vi "lanelog2.vi"(6 "xsensor":T1={"idx"=1, "x"=-35.60561147, "y"=-90.69379038, "h"=0.8330275943157105, "x_path"=0.0}, 7 "thresh":dbl=0.02, 8 "lane_log":dbl[][](array[numeric])=array7715x4[30860 elements], 9 "sensor":dbl[][](array[numeric])=[[-3.0874260564438702, 8.254219212686142, 0.33125647926136603, -1.2, 268.0], [-3.251465137645852, 8.1435734553204, 0.33125647926136603, -1.2, 284.0], [-3.2918636404136175, 8.115022616326533, 0.33125647926136603, -1.2, 272.0], [-3.2146540135510326, 8.265920567763587, 0.3295810856706975, -1.2, 268.0], [-3.0941669932632254, 8.356869302518275, 0.3293716614718639, -1.2, 216.0], [-3.0675596258112376, 8.409121589077968, 0.32874338887536325, -1.2, 248.0], [-3.1950142718158414, 8.327140005961258, 0.32874338887536325, -1.2, 236.0], [-3.278772864980552, 8.270644121512921, 0.32874338887536325, -1.2, 248.0], [-2.9865656875850273, 8.47047999653983, 0.3285339646765297, -1.2, 232.0], [-3.035050878170219, 8.452752896063785, 0.3283245404776961, -1.2, 204.0], [-2.9543519196681682, 8.617087628303914, 0.32623029848936036, -1.2, 224.0], [-2.998893873836392, 8.591111528384989, 0.32623029848936036, -1.2, 196.0], [-2.9033727279755284, 8.737823052620522, 0.3245549048986918, -1.2, 216.0], [-2.968662847780547, 8.747093819694697, 0.3237172081033576, -1.2, 192.0], [-2.9052595387814195, 8.85082243489861, 0.32246066291035613, -1.2, 188.0], [-2.734592721427704, 8.98474447764757, 0.32162296611502184, -1.2, 204.0], [-2.791429232542248, 8.978488337161597, 0.3212041177173547, -1.2, 224.0], [-2.839131166422159, 8.953920226823765, 0.3212041177173547, -1.2, 196.0], [-2.886616889471603, 8.928936779344951, 0.3212041177173547, -1.2, 216.0], [-2.6987125748878515, 9.157968574659893, 0.3186910273313519, -1.2, 196.0], [-2.765515279987869, 9.17014660250537, 0.3178533305360176, -1.2, 220.0], [-2.6830373985326297, 9.253792269139186, 0.3170156337406833, -1.2, 220.0], [-4.28548337639476, 9.508026110543323, 0.39847829900104376, -0.3999999999999999, 204.0], [6.270261138102536, 8.950654849997015, 0.2759684907693037, -1.2, 308.0], [6.263336924153402, 9.139533897307718, 0.27345540038330085, -1.2, 304.0], [6.193207282056716, 9.275259222095512, 0.27261770358796655, -1.2, 312.0], [6.091471855365504, 9.38246599277969, 0.27261770358796655, -1.2, 324.0], [6.4696355580106255, 9.02559077208453, 0.2717800067926323, -1.2, 240.0], [6.372215345218233, 9.137659907105647, 0.2717800067926323, -1.2, 256.0], [6.331823345079176, 9.30204711946733, 0.2701046132019638, -1.2, 264.0], [6.072715111455862, 9.572715111455864, 0.2701046132019638, -1.2, 332.0], [6.258607904594664, 9.439197138421996, 0.2692669164066295, -1.2, 276.0], [6.182525166787418, 9.57555056054587, 0.2684292196112952, -1.2, 276.0], [6.049147437675454, 9.764075544301484, 0.2675915228159609, -1.2, 328.0], [6.0207247852542345, 9.956436871376717, 0.2650784324299581, -1.2, 324.0], [6.215701669208983, 9.825143971096239, 0.2642407356346238, -1.2, 276.0], [6.104366004380429, 9.932659572856856, 0.2642407356346238, -1.2, 280.0], [6.045206253694134, 10.097184975373532, 0.2625653420439552, -1.2, 284.0], [5.987405501886605, 10.149687481752428, 0.2625653420439552, -1.2, 332.0], [6.008645752931635, 10.291538564175015, 0.2600522516579524, -1.2, 288.0], [5.949150359744033, 10.34371462365704, 0.2600522516579524, -1.2, 332.0], [5.967118589360381, 10.48659821129467, 0.2575391612719496, -1.2, 292.0], [5.905922582465032, 10.538404455235977, 0.2575391612719496, -1.2, 332.0], [5.845104223695827, 10.718102585492996, 0.25544491928361385, -1.2, 344.0], [5.742861784006737, 10.85052788528084, 0.2546072224882796, -1.2, 352.0], [5.946027011549364, 10.713107553966188, 0.25418837409061246, -1.2, 296.0], [5.685904682379038, 11.045450364978343, 0.2520941321022767, -1.2, 352.0], [5.893920691194497, 10.90967382499498, 0.2516752837046096, -1.2, 296.0], [5.812396612769266, 11.074862742777189, 0.24999989011394105, -1.2, 300.0], [5.635624312811938, 11.256771414722133, 0.24916219331860678, -1.2, 340.0], [5.750674853192741, 11.271591029935388, 0.24748679972793824, -1.2, 300.0], [5.545267703886312, 11.419463018156659, 0.24748679972793824, -1.2, 340.0], [5.462116471720623, 11.597920686443521, 0.24539255773960256, -1.2, 344.0], [5.683835103994589, 11.468442930129942, 0.24497370934193538, -1.2, 284.0], [5.566552204276135, 11.599383715798275, 0.2441360125466011, -1.2, 284.0], [5.51264120473925, 11.828692341891706, 0.240785225365264, -1.2, 288.0], [5.439750670877296, 11.876481469970823, 0.240785225365264, -1.2, 336.0], [5.303328472257424, 11.987099673000078, 0.24036637696759688, -1.2, 344.0], [-1.928655864366284, 13.422074272450256, 0.2382721349792612, -1.2, 324.0], [5.216191450902815, 12.181200407749735, 0.23785328658159402, -1.2, 348.0], [5.473882232873657, 12.092273991781463, 0.23659674138859263, -1.2, 284.0], [5.323092676171175, 12.186497764352836, 0.23659674138859263, -1.2, 296.0], [5.153869423312828, 12.426763696753529, 0.23408365100258977, -1.2, 340.0], [5.2721670641556875, 12.450363583742815, 0.2324082574119212, -1.2, 288.0], [-1.900299672338241, 13.75309951845401, 0.23157056061658696, -1.2, 296.0], [-1.8211698834585328, 13.82836765049368, 0.2303140154235855, -1.2, 372.0], [5.174236572168083, 12.645432179932216, 0.2298951670259184, -1.2, 288.0], [5.103925680397715, 12.70772566679367, 0.22947631862825127, -1.2, 344.0], [5.017550333081534, 12.936639702633745, 0.22612553144691414, -1.2, 344.0], [5.147413862635719, 12.980356990567492, 0.22403128945857842, -1.2, 288.0], [8.180852483152144, 10.611506567635107, 0.3743231383700968, -0.3999999999999999, 264.0], [4.942872250794322, 13.200933006778827, 0.22193704747024273, -1.2, 348.0], [5.055038418263844, 13.210638452637436, 0.2206805022772413, -1.2, 288.0], [-1.8068749197163638, 14.297458756228902, 0.2206805022772413, -1.2, 308.0], [8.174393871184286, 10.860257301297807, 0.373206136722423, -0.3999999999999999, 256.0], [8.132454974984348, 11.083636951508186, 0.37236838548666756, -0.3999999999999999, 264.0], [4.974014493298352, 13.47632967793971, 0.21649201830056994, -1.2, 288.0], [4.886766302989657, 13.51935572391995, 0.21649201830056994, -1.2, 308.0], [8.02763653917211, 11.252198494109617, 0.3720891350747491, -0.3999999999999999, 284.0], [8.41805715455429, 10.9476678431101, 0.37153063425091215, -0.3999999999999999, 212.0], [-1.762629762368157, 14.628806331963263, 0.2139789279145671, -1.2, 312.0], [8.004253700261659, 11.50425370026166, 0.37097213342707525, -0.3999999999999999, 304.0], [8.353148660757368, 11.154250519053866, 0.37090232082409563, -0.3999999999999999, 220.0], [8.218291344725634, 11.298867285084208, 0.37090232082409563, -0.3999999999999999, 236.0], [8.622793513388025, 10.864561394524376, 0.370832508221116, -0.3999999999999999, 176.0], [7.974483755589461, 11.757819665743355, 0.36985513177940144, -0.3999999999999999, 320.0], [8.202180279054376, 11.560260111808223, 0.3697155065734422, -0.3999999999999999, 248.0], [4.954095970806885, 13.886478196863694, 0.20895274714256143, -1.2, 248.0], [4.880170386307381, 13.965559166701984, 0.20811505034722713, -1.2, 260.0], [7.945087273837262, 12.020062990878387, 0.36866831752874796, -0.3999999999999999, 368.0], [8.263518845062517, 11.909017868700095, 0.3676909410870333, -0.3999999999999999, 256.0], [8.115502673534229, 12.051955424034883, 0.3676909410870333, -0.3999999999999999, 296.0], [-1.7422907602406512, 15.157939689347018, 0.20308886957522146, -1.2, 264.0], [7.929004456398092, 12.306051579412163, 0.36727206546915564, -0.3999999999999999, 392.0], [7.774110039342803, 12.443090583519641, 0.36727206546915564, -0.3999999999999999, 412.0], [4.917183201802519, 14.28977377780451, 0.20162290018338652, -1.2, 224.0], [8.052839027989592, 12.288131688987452, 0.36678337724829835, -0.3999999999999999, 348.0], [4.891968691273311, 14.487541577387939, 0.19806268880321581, -1.2, 260.0], [7.771112819957454, 12.761251621639218, 0.36559656299764487, -0.3999999999999999, 416.0], [8.030759275666764, 12.57712212750872, 0.365387125188706, -0.3999999999999999, 360.0], [-1.6961480258098567, 15.568720307529205, 0.19471190162187874, -1.2, 296.0], [7.949050394089805, 12.807142204926757, 0.3645493739529506, -0.3999999999999999, 372.0], [7.7089869232088795, 13.01980603123654, 0.364479561349971, -0.3999999999999999, 424.0], [7.566295141983507, 13.184416153684932, 0.36420031093805255, -0.3999999999999999, 448.0], [4.907524501146654, 14.786533649341463, 0.19219881123587584, -1.2, 304.0], [7.938062739362771, 13.129640127422718, 0.36287387148143985, -0.3999999999999999, 380.0], [7.76879334061014, 13.266711783841115, 0.36287387148143985, -0.3999999999999999, 396.0], [7.516486463232196, 13.474714437812196, 0.36280405887846023, -0.3999999999999999, 456.0], [4.902600205433592, 15.049802292658747, 0.18717263046387017, -1.2, 300.0], [7.411791406878046, 13.701455690730548, 0.3619663076427049, -0.3999999999999999, 468.0], [7.6945569471755055, 13.527741846330688, 0.361756869833766, -0.3999999999999999, 424.0], [7.278507600876223, 13.894786122248709, 0.3614078068188679, -0.3999999999999999, 480.0], [7.5659614658398775, 13.724810089569369, 0.3611983690099291, -0.3999999999999999, 432.0], [7.163086529840346, 14.119712503220669, 0.36057005558311256, -0.3999999999999999, 492.0], [-1.6742837675349664, 16.217447813122682, 0.18130875289653026, -1.2, 288.0], [7.456044248361615, 13.952988517530661, 0.3603606177741737, -0.3999999999999999, 440.0], [4.939359591017299, 15.424668914071585, 0.17963335930586166, -1.2, 276.0], [7.340445944696752, 14.180415124015806, 0.3595228665384183, -0.3999999999999999, 456.0], [4.910015355954023, 15.652714457593937, 0.1754448753291903, -1.2, 272.0], [-2.0742704566937493, 16.596428237795855, 0.35742848844902986, -0.3999999999999999, 244.0], [7.351621486160834, 14.60708847142727, 0.3570096128311522, -0.3999999999999999, 460.0], [-1.6314726207982264, 16.787278211536382, 0.16958099776185032, -1.2, 292.0], [6.947694316000941, 15.062905099763684, 0.3558227985804987, -0.3999999999999999, 576.0], [4.950345642278116, 16.06718454758031, 0.16706790737584754, -1.2, 240.0], [7.3285880609769, 15.003578979950875, 0.35477560953580445, -0.3999999999999999, 476.0], [4.940810185204615, 16.371250584204297, 0.16120402980850757, -1.2, 248.0], [7.377499944938261, 15.538985731940056, 0.3514246045927829, -0.3999999999999999, 480.0], [4.971854164908072, 16.797828014132726, 0.15261763765633118, -1.2, 220.0], [4.975301680149189, 17.169529021184545, 0.14528779069715625, -1.2, 228.0], [-1.5383215259591212, 18.136151645750907, 0.1417275793169856, -1.2, 172.0], [1.6829626062501868, 18.271173220882176, 0.13858621633448204, -1.2, 76.0], [4.982643392608833, 17.570550880741774, 0.13732967114148065, -1.2, 208.0], [-1.1993764728960121, 18.73952302036782, 0.12979039998347214, -1.2, 436.0], [4.9833552728263575, 17.972714590665475, 0.129371551585805, -1.2, 192.0], [1.621925956717769, 18.9315946699765, 0.12497364341030004, -1.2, 236.0], [-1.4948658186201547, 19.024775107896094, 0.1232982498196315, -1.2, 172.0], [4.9710734881443015, 18.356972582706735, 0.12183228042779648, -1.2, 184.0], [10.1762046864033, 15.52061845794352, 0.5599548496928946, 0.40000000000000013, 412.0], [4.4892978065922735, 18.655615402218494, 0.1189003416441265, -1.2, 392.0], [10.116711660579657, 15.882236625148431, 0.5616303521644053, 0.40000000000000013, 432.0], [4.423009309038194, 18.924866549582596, 0.11387416087212082, -1.2, 424.0], [4.9679034872117604, 18.789634776867167, 0.1132458882756201, -1.2, 180.0], [10.208563049778917, 16.21960594386651, 0.563864355459753, 0.40000000000000013, 388.0], [-1.4211984035446172, 19.7443720851159, 0.10842913170244806, -1.2, 224.0], [4.9154615434653435, 19.08985228247094, 0.1075914349071137, -1.2, 216.0], [4.802613585016308, 19.208641220118103, 0.10591604131644522, -1.2, 268.0], [-1.86214748615549, 19.843858727865292, 0.3351582680985325, -0.3999999999999999, 500.0], [4.41648153671134, 19.425317939974306, 0.10382179932810948, -1.2, 440.0], [10.245755173166765, 16.496678478471168, 0.5655398579312637, 0.40000000000000013, 396.0], [10.13194907010119, 16.585593551005047, 0.5655398579312637, 0.40000000000000013, 424.0], [8.89513720681148, 17.59793922259855, 0.5663776091670192, 0.40000000000000013, 364.0], [-1.803072050702221, 20.655084627603436, 0.3295732598601633, -0.3999999999999999, 420.0], [-1.4600881893088467, 22.052179466228814, 0.32007874585493556, -0.3999999999999999, 508.0], [-1.6254149910617555, 22.078578361528226, 0.3197994954430171, -0.3999999999999999, 368.0], [-0.876993498557809, 23.58645347846649, 0.02884793614569159, -1.2, 264.0], [-1.7323054850638269, 24.34764225753624, 0.5960479654333557, 0.40000000000000013, 184.0], [4.576693870008543, 24.144131958105543, 0.0070678194670003025, -1.2, 164.0], [-1.7766743936812326, 24.881605315546707, 0.8994243306968406, 1.2000000000000006, 212.0], [-15.383269013420207, 18.88326901342021, -0.005707056661847398, -1.2, 172.0], [-15.516925908799797, 18.748440622546504, -0.005707056661847398, -1.2, 176.0], [-15.663784770939868, 18.62634112429063, -0.006125905059514547, -1.2, 156.0], [-15.867710423236526, 18.557894946543833, -0.00822014704785018, -1.2, 132.0], [1.9091635206414816, 25.321838895456125, -0.008848419644350902, -1.2, 340.0], [-15.161125487767853, 19.4764927159004, -0.011361510030353794, -1.2, 164.0], [-1.6392398550297682, 25.55863652788837, 0.6044254777909096, 0.40000000000000013, 188.0], [4.639571181211605, 25.327466274196635, -0.017434811796527283, -1.2, 172.0], [-0.7857642968418002, 26.001345425033872, -0.02162329577319866, -1.2, 236.0], [0.19726369493970786, 26.104180522661046, -0.023508113562700772, -1.2, 208.0], [3.9287964216078732, 25.781311718843845, -0.02392696196036792, -1.2, 224.0], [-1.6774482452010537, 26.072792518250637, 0.9241363861592018, 1.2000000000000006, 220.0], [1.1851494290302318, 26.1139982507089, -0.024345810358035125, -1.2, 212.0], [2.989699229479819, 26.209020218132554, -0.02979083952770789, -1.2, 252.0], [2.7914143198272865, 26.23424524468249, -0.02979083952770789, -1.2, 116.0], [-0.0, 26.424971072078208, -0.03020968792537504, -1.2, 84.0], [5.3831189045097885, 25.922303935324, 0.2890121375290067, -0.3999999999999999, 244.0], [-1.5343200205313599, 26.909199859587602, 0.6137803665901781, 0.40000000000000013, 200.0], [4.702058107639062, 26.6113539682675, -0.04403168504839061, -1.2, 160.0], [-1.5981019113415127, 27.882323464453414, 0.9618327419492443, 1.2000000000000006, 180.0], [16.87235585354733, 21.43584249865242, 0.965811801727082, 1.2000000000000006, 236.0], [-0.6472139558002346, 28.216103807544194, -0.06790604371541759, -1.2, 80.0], [16.912004682939006, 21.79530359253437, 0.9718851034932556, 1.2000000000000006, 276.0], [4.761548009355336, 27.996040933764434, -0.07272280028858963, -1.2, 136.0], [16.966816300178685, 22.179008023982007, 0.97858667785593, 1.2000000000000006, 252.0], [17.14934975532431, 22.71422306055236, 0.9894767361952754, 1.2000000000000006, 192.0], [17.0667193182793, 22.960863590383795, 0.9921992507801118, 1.2000000000000006, 72.0], [5.438837287934404, 29.087717665370338, 0.26737023060532583, -0.3999999999999999, 140.0], [5.5183699426079125, 30.623654823461283, 0.2567587149524243, -0.3999999999999999, 136.0], [5.594383409940466, 32.280607638486906, 0.24530944806376734, -0.3999999999999999, 136.0], [2.3560692275628514, 33.43669797801458, 0.24035275325221464, -0.3999999999999999, 200.0], [5.663742107532391, 34.05881781210548, 0.23302242993935499, -0.3999999999999999, 128.0], [15.696846843198209, 30.963785907053047, 1.1126181651094145, 1.2000000000000006, 216.0], [15.945986127827634, 30.8430340000858, 1.1130370135070815, 1.2000000000000006, 212.0], [15.47612601588197, 31.13461144760037, 1.1134558619047488, 1.2000000000000006, 220.0], [-1.573164496371527, 36.25144044389028, 0.6789155251701594, 0.40000000000000013, 176.0], [-1.2951497592364731, 36.463762582363366, 0.6803117772297517, 0.40000000000000013, 180.0], [5.758033248807259, 36.15542928071491, 0.21850140851959496, -0.3999999999999999, 128.0], [10.0910638783173, 35.998536724162264, 0.6875722879396318, 0.40000000000000013, 264.0], [-0.8195652580345191, 41.06014402087102, 0.7122859493944156, 0.40000000000000013, 236.0], [6.04917334542589, 41.692977372214614, 0.18003466427782683, -0.3999999999999999, 120.0], [6.247751551440067, 45.30468176887548, 0.15490212720516522, -0.3999999999999999, 84.0], [10.576764453944458, 46.723668750702885, 0.7606660832592892, 0.40000000000000013, 160.0], [18.29351193435394, 44.11009062363429, 1.382984805803553, 1.2000000000000006, 164.0], [10.286262869518918, 47.1841965407068, 0.7633189621725146, 0.40000000000000013, 148.0], [6.550718221917733, 50.11078209610396, 0.12139207777494981, -0.3999999999999999, 40.0], [10.924256810644076, 51.77826832915608, 0.795572384749097, 0.40000000000000013, 160.0], [-1.7372882317377514, 18.747983116378037, 0.12853385479047075, -1.2, 120.0], [11.262063566611518, 15.06083163069632, 0.5626775412090995, 0.40000000000000013, 100.0], [8.976613577038671, 17.86558466119368, 0.33173745055253134, -0.3999999999999999, 160.0], [8.96290906479165, 18.71600016117027, 0.32671094313799903, -0.3999999999999999, 164.0], [-2.155816147837948, 21.05771354301394, 0.3265015053290602, -0.3999999999999999, 380.0], [9.024780067116186, 19.131377603380102, 0.323988251621794, -0.3999999999999999, 156.0], [9.045600358828692, 19.48804450755426, 0.3217542483264463, -0.3999999999999999, 148.0], [9.041479077757348, 19.811260034561684, 0.3197994954430171, -0.3999999999999999, 156.0], [-1.3236875014373035, 22.42961318623577, 0.05251287061388493, -1.2, 156.0], [9.07056698382929, 20.205906190633105, 0.31728624173575093, -0.3999999999999999, 156.0], [9.093442564981476, 20.602278093067493, 0.31477298802848475, -0.3999999999999999, 152.0], [5.027751135547025, 22.263822685673617, 0.04308878166637431, -1.2, 220.0], [13.677266938894665, 19.945126022164064, 0.5993291577733977, 0.40000000000000013, 108.0], [6.320922215936061, 24.174804981229045, 0.2990651523580713, -0.3999999999999999, 168.0], [-1.5122834965924712, 25.12666157030228, 0.2986462767401936, -0.3999999999999999, 292.0], [-15.18884666612654, 19.228511154290864, -0.00801072284901666, -1.2, 164.0], [-15.991197551190128, 18.41203296189243, -0.00801072284901666, -1.2, 124.0], [4.974826021189758, 25.048338889544475, -0.013246327819855908, -1.2, 136.0], [-15.18477247651323, 19.783674872656796, -0.01638769080235941, -1.2, 164.0], [-15.143410526013682, 20.02613264222062, -0.019529053784863026, -1.2, 152.0], [6.004699976609632, 25.15224862071348, 0.29313108110480396, -0.3999999999999999, 64.0], [-15.132414799181563, 20.306249255557532, -0.023717537761534402, -1.2, 152.0], [5.8672847673986706, 25.397004854406784, 0.29173482904521164, -0.3999999999999999, 120.0], [-14.882714626526145, 20.620604720041705, -0.025183507153369367, -1.2, 212.0], [-15.03791801192453, 21.107139779497775, -0.03502644449854714, -1.2, 176.0], [0.41091403159128786, 27.04124910340555, -0.04319398825305637, -1.2, 120.0], [3.8942692333612956, 26.7712353102285, -0.044241109247224186, -1.2, 92.0], [1.0339888538441397, 27.182238288137274, -0.04654477543439345, -1.2, 116.0], [3.756731756174191, 27.219070815772636, -0.053036925598234086, -1.2, 96.0], [16.668723246512226, 20.91237546586442, 0.9549217433877364, 1.2000000000000006, 160.0], [-15.042878891887115, 22.411490638873143, -0.056178288580737645, -1.2, 148.0], [0.6330815038741477, 27.676407242397655, -0.056597136978404794, -1.2, 112.0], [3.3978617547396803, 27.677042650522004, -0.06141389355157695, -1.2, 152.0], [-15.049621716930838, 22.76263738425686, -0.062042166148077615, -1.2, 148.0], [0.8538033900408014, 27.949730131020374, -0.062461014545744764, -1.2, 116.0], [3.6294029746828156, 27.784902355416687, -0.06434583233524688, -1.2, 88.0], [-15.051368401443346, 23.115325196741345, -0.06790604371541759, -1.2, 144.0], [16.331597840810588, 22.122618200125487, 0.6229258175805077, 0.40000000000000013, 156.0], [5.625888766858202, 27.868401465052543, 0.2753986799479816, -0.3999999999999999, 100.0], [-15.066143200716514, 23.4934473163024, -0.07439819387925822, -1.2, 132.0], [-15.224123706487509, 24.074222375009924, -0.08612594901393816, -1.2, 132.0], [15.388533709826934, 24.10774585394575, 0.6295580148635712, 0.40000000000000013, 60.0], [-15.18503985850474, 24.40041432288007, -0.09115212978594373, -1.2, 92.0], [15.450544583691912, 24.57188399004637, 0.6324203315857354, 0.40000000000000013, 88.0], [9.403345837579257, 27.9965534130117, 0.2668117297814889, -0.3999999999999999, 128.0], [5.703044844702137, 29.224772877763986, 0.2660437911487131, -0.3999999999999999, 64.0], [9.466886860277452, 29.510057881143965, 0.2567587149524243, -0.3999999999999999, 128.0], [15.599171906131094, 29.719850640073204, 0.6629982516908071, 0.40000000000000013, 176.0], [15.848136819476986, 29.6169211826018, 0.6632775021027255, 0.40000000000000013, 176.0], [16.228041929851543, 29.72422353746002, 0.6653020675891343, 0.40000000000000013, 148.0], [-1.0867438434896055, 34.62027195581754, 0.2326035543214773, -0.3999999999999999, 208.0], [11.202409620014603, 33.06825475520069, 0.6707474506215444, 0.40000000000000013, 132.0], [10.995870935203495, 33.30561238280741, 0.6717946396662386, 0.40000000000000013, 88.0], [10.418705939012487, 35.09571994456489, 0.682266530113181, 0.40000000000000013, 104.0], [5.888755068804653, 38.68981269103743, 0.20090863256873187, -0.3999999999999999, 128.0], [21.264902026527764, 37.86369875407095, 1.2964926116852886, 1.2000000000000006, 108.0], [21.17311499265992, 39.08880663879596, 1.3174350315686456, 1.2000000000000006, 84.0], [21.513995338753997, 38.95396704895709, 1.3186915767616472, 1.2000000000000006, 124.0], [17.080070877486495, 42.31741385340898, 0.7460752492365496, 0.40000000000000013, 156.0], [8.278950878194507, 19.403716667083884, 0.32482600285754937, -0.3999999999999999, 48.0], [-2.667894854589383, 21.35130129946067, 0.323988251621794, -0.3999999999999999, 340.0], [8.149121025638326, 20.208174144360875, 0.3202183710608948, -0.3999999999999999, 124.0], [9.120446875494231, 21.399884852746606, 0.3097464806139525, -0.3999999999999999, 152.0], [6.279426242486466, 24.69898772096905, 0.2956443348120701, -0.3999999999999999, 84.0], [9.243287120931221, 23.78254244454064, 0.29438770795843705, -0.3999999999999999, 148.0], [6.229252435277006, 25.223984917116187, 0.292223517266069, -0.3999999999999999, 60.0], [9.244898599965028, 24.264382226537055, 0.29131595342733396, -0.3999999999999999, 144.0], [-15.084549481174566, 20.549981599367705, -0.026858900744037906, -1.2, 148.0], [9.334488223102976, 24.967853172167995, 0.2865686964247201, -0.3999999999999999, 152.0], [16.333140340768534, 20.56182098917662, 0.6148973682378519, 0.40000000000000013, 100.0], [16.27269945637997, 20.798388974896767, 0.6158049320765869, 0.40000000000000013, 108.0], [11.633788245920316, 24.27362367751091, 0.6162238076944646, 0.40000000000000013, 120.0], [9.318710318537917, 25.453505750353774, 0.283496941893617, -0.3999999999999999, 144.0], [16.270457361193163, 21.101281609903406, 0.6173408093421384, 0.40000000000000013, 120.0], [16.223815690819396, 21.36102814499319, 0.6184578109898123, 0.40000000000000013, 124.0], [9.306634273479593, 25.968202683080712, 0.2802157495535751, -0.3999999999999999, 136.0], [16.213823438051257, 21.66605437803303, 0.6199936882553638, 0.40000000000000013, 136.0], [7.840406989925826, 26.93250647257559, 0.2774930580373701, -0.3999999999999999, 84.0], [8.09993828830126, 27.023928885387402, 0.27630624378671664, -0.3999999999999999, 92.0], [16.377343075265326, 22.506842263569443, 0.6251598208758554, 0.40000000000000013, 112.0], [7.736971672108107, 28.038539141289487, 0.2703721725334493, -0.3999999999999999, 76.0], [16.245694733302315, 24.864173105513157, 0.6373770263972881, 0.40000000000000013, 84.0], [9.529953587218, 30.411758734122486, 0.25068501849319774, -0.3999999999999999, 120.0], [14.563985000188746, 30.04663922418586, 0.6613925618222759, 0.40000000000000013, 188.0], [15.284129991017839, 29.70813053868281, 0.6618114374401536, 0.40000000000000013, 204.0], [15.084614101362881, 29.892600775732266, 0.6622303130580313, 0.40000000000000013, 188.0], [-1.3574022550676748, 34.58962300498183, 0.23274317952743653, -0.3999999999999999, 92.0], [9.62873489352778, 33.13419886563537, 0.23246392911551808, -0.3999999999999999, 88.0], [15.941280736440438, 32.55711784764017, 1.1442412191332834, 1.2000000000000006, 112.0], [-0.9436559897075923, 39.536768353342815, 0.19832556625848607, -0.3999999999999999, 76.0], [-0.6715522340536157, 41.97320172198243, 0.18136110373443953, -0.3999999999999999, 132.0], [-0.3541141808009181, 44.077465969623496, 0.16670045710872028, -0.3999999999999999, 104.0], [17.438697502854822, 42.21247295163448, 0.7464243122514476, 0.40000000000000013, 164.0], [17.80935122293895, 42.131469169923385, 0.7469828130752845, 0.40000000000000013, 160.0]], 11 "Lane_M":dbl[](array[numeric])=[0.8601491478953653, 0.8717844136967624, 0.882947592858927, 0.8936326403234123, 0.9038337699485205, 0.9135454576426009, 0.9227624443554423, 0.9314797389261423, 0.9396926207859084, 0.9473966425143293, 0.9545876322477319, 0.9612616959383189, 0.9674152194628639, 0.9730448705798238, 0.9781476007338057, 0.9827206467064133, 0.9867615321125792, 0.9902680687415704, 0.993238357741943, 0.9956707906498045, 0.9975640502598242, 0.9989171113385246, 0.9997292411794617, 1.0, 0.9997292411794617, 0.9989171113385246, 0.9975640502598242, 0.9956707906498045, 0.993238357741943, 0.9902680687415704, 0.9867615321125792, 0.9827206467064133]) -> (0 "lane_log_out":dbl[][](array[numeric]), 1 "sensor_out":dbl[][](array[numeric]), 2 "lane_I_out":dbl[](array[numeric]), 3 "lane_M_out":dbl[](array[numeric]), 4 "size":i32)   [LabVIEW 2012]
uses:
  G_NAV.vi
  G_SEN.vi
  <vilib>/Analysis/Matrix/Numeric/Conversions/Array To Matrix - RA2.vi
  <vilib>/Analysis/baseanly.llb/Real Inverse Matrix.vi
  <vilib>/Analysis/baseanly.llb/A x Vector.vi
  <vilib>/Analysis/NI_AALBase.lvlib
  <vilib>/Analysis/Matrix/NI_Matrix.lvlib
panel:
  out "Y":dbl[](array[numeric])
  out "X":dbl[](array[numeric])
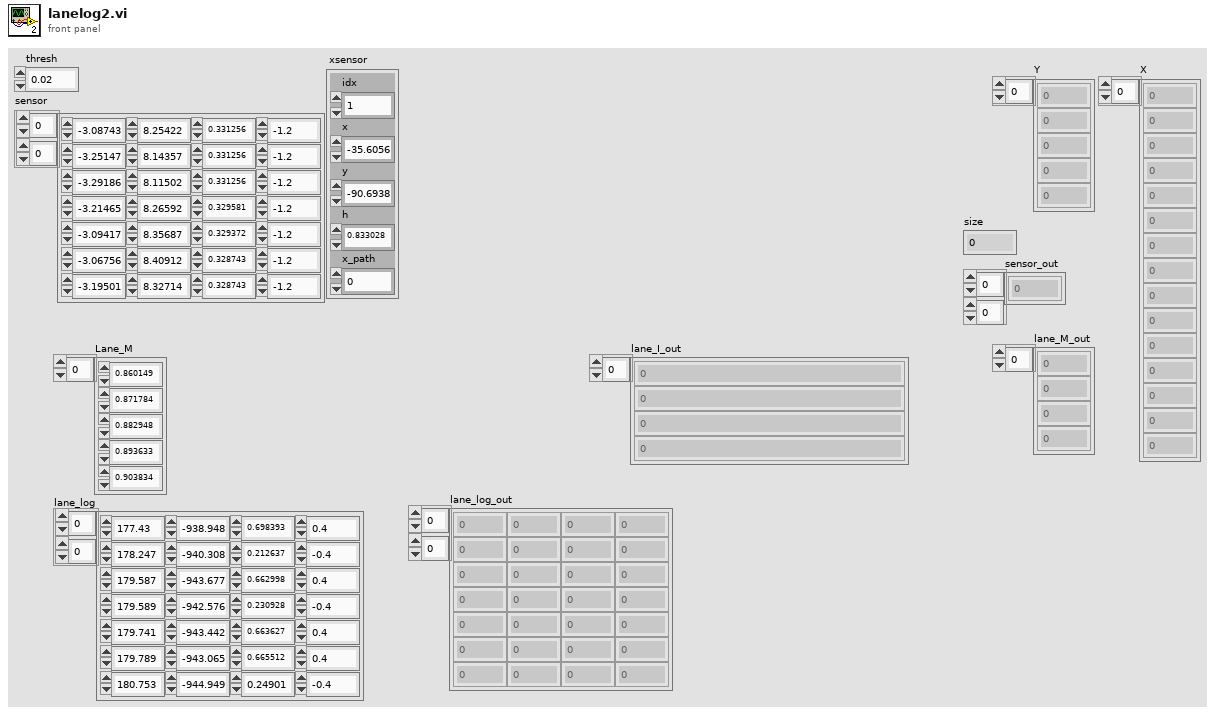
[diagram p1: front panel]
types:
  T1 = cluster{"idx":i32, "x":dbl, "y":dbl, "h":dbl, "x_path":dbl}
  T2 = cluster{"GPSTime":dbl, "attitude[2]":dbl, "lcc[0]":dbl, "lcc[1]":dbl, "heading_GPS":dbl}
  T3 = cluster{i16, "element":dbl, "element":dbl, "element":dbl, "element":dbl}[]
  T4 = cluster{i16, "Real Matrix Element":dbl, "Real Matrix Element":dbl}[]
  T5 = typedef "NI_Matrix.lvlib/RealMatrix.ctl" = dbl[][]
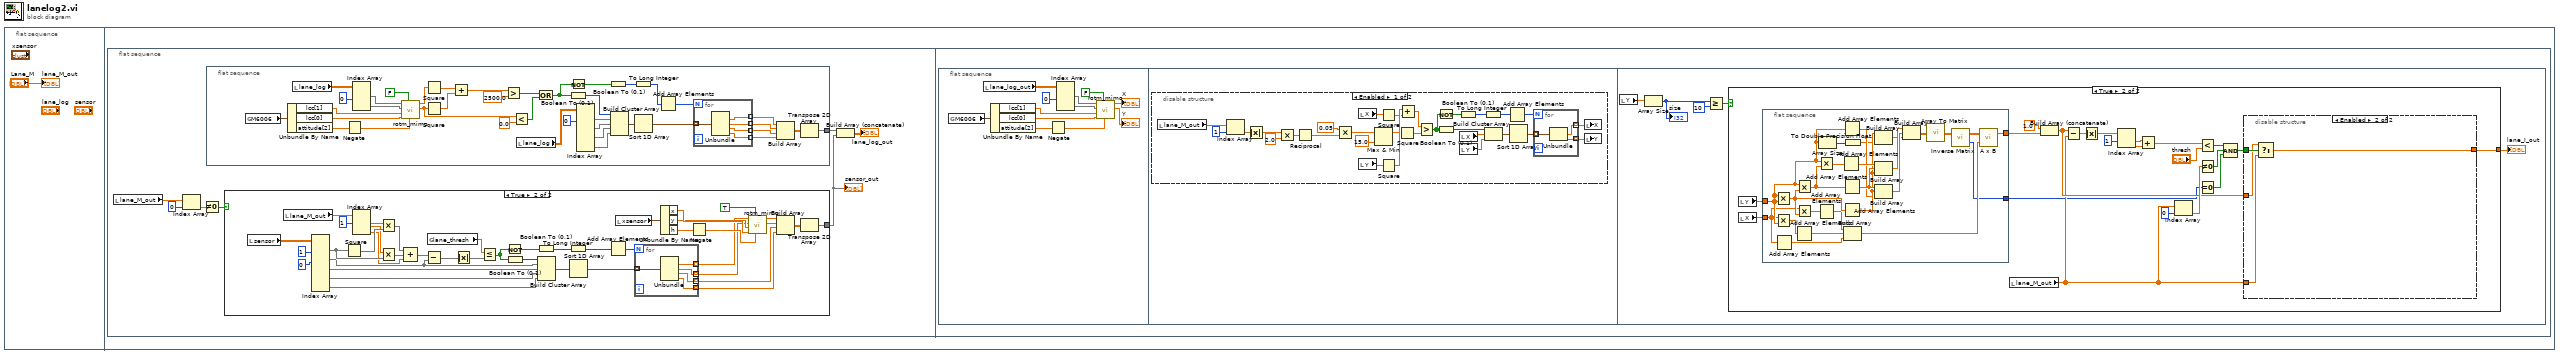
[diagram p0: block diagram]
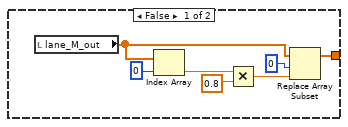
[diagram p4: hidden frame]
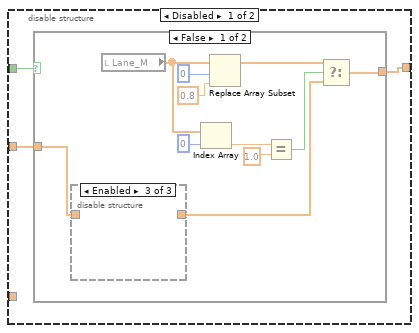
[diagram p5: hidden frame]
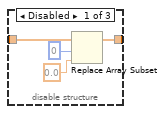
[diagram p6: hidden frame]
diagram:
  n1 = flat-sequence {
    frame #0 {
      "lane_M_out" <- "Lane_M"
    }
    frame #1 {
      n2 = flat-sequence {
        frame #0 {
          n3 = local read "lane_M_out"() -> (w6:dbl[])
          n4 = Index Array(array=w6, index=0) -> (element=w4:dbl)
          n5 = Not Equal To 0?(x=w4) -> (x != 0?=w3:bool)
          n6 = flat-sequence {
            tunnel: [w94] -> w8
            frame #0 {
              n7 = global read "G_NAV.vi" "M6006"() -> (w59:T2)
              n8 = Unbundle By Name(w59) -> ("lcc[1]"=w58:dbl, "lcc[0]"=w57:dbl, "attitude[2]"=w56:dbl)
              n9 = local read "lane_log"() -> (w71:dbl[][])
              n10 = Negate(x=w56) -> (-x=w92:dbl)
              n11 = Index Array(array=w71, index (col) #1=0 ("disabled index (col)")) -> (element #1=w90:dbl[], element #2=w89:dbl[])  [unwired: 3 in]
              n12 = call "rotm_mimo.vi"("angle[rad]"=w92, "reverse"=FALSE, "y0"=w57, "x0"=w58, "y"=w89, "x"=w90) -> ("Y"=w68:dbl[], "X"=w67:dbl[])  [unwired: 2 in, 2 out]
              n13 = Square(x=w67) -> (x^2=w65:dbl[])
              n14 = Square(x=w68) -> (x^2=w66:dbl[])
              n15 = Add(x=w65, y=w66) -> (x+y=w64:dbl[])
              n16 = Greater?(x=w64, y=2500.0) -> (0:w62:bool[])
              n17 = Less?(x=w68, y=0.0) -> (x < y?=w61:bool[])
              n18 = local read "lane_log"() -> (w70:dbl[][])
              n19 = Or(x=w62, y=w61) -> (x .or. y?=w60:bool[])
              n20 = Not(x=w60) -> (.not. x?=w85:bool[])
              n21 = Boolean To (0,1)(Boolean=w60) -> (0, 1=w88:i16[])
              n22 = Index Array(array=w70, index (col) #1=0 ("disabled index (col)")) -> (element #1=w83:dbl[], element #2=w82:dbl[], element #3=w81:dbl[], element #4=w80:dbl[])  [unwired: 7 in]
              n23 = Boolean To (0,1)(Boolean=w85) -> (0, 1=w86:i16[])
              n24 = Build Cluster Array(w88, w83, w82, w81, w80) -> (w78:T3)
              n25 = To Long Integer(number=w86) -> (32bit integer=w87:i32[])
              n26 = Sort 1D Array(array=w78) -> (sorted array=w77:T3)
              n27 = Add Array Elements(numeric array=w87) -> (sum=w79:i32)
              n28 = for {
                N: w79 -> [_]
                tunnel: w77 -> [w99] mode=indexing
                tunnel: [w98] -> w76 mode=indexing
                tunnel: [w97] -> w75 mode=indexing
                tunnel: [w96] -> w74 mode=indexing
                tunnel: [w95] -> w73 mode=indexing
                n29 = Unbundle(w99) -> ("element"=w98:dbl, "element"=w97:dbl, "element"=w96:dbl, "element"=w95:dbl)  [unwired: 1 out]
              }
              n30 = Build Array(w76, w75, w74, w73) -> (w72:dbl[][])
              n31 = Transpose 2D Array(2D array=w72) -> (transposed array=w94:dbl[][])
            }
          }
          n32 = case shown="True" w3 {
            tunnel: [_ w50] -> w2
            frame False {
            }
            frame True {
              n33 = local read "sensor"() -> (w10:dbl[][])
              n34 = local read "lane_M_out"() -> (w11:dbl[])
              n35 = Index Array(array=w10, index (col) #1=1 ("disabled index (col)"), index (col) #2=0 ("index (col)")) -> (element #1=w45:dbl[], element #2=w34:dbl[], element #3=w33:dbl[], element #4=w32:dbl[], element #5=w31:dbl[])  [unwired: 8 in]
              n36 = Square(x=w45) -> (x^2=w47:dbl[])
              n37 = Index Array(array=w11, index #1=1 ("index")) -> (element #1=w46:dbl, element #2=w44:dbl, element #3=w41:dbl)  [unwired: 2 in]
              n38 = Multiply(x=w46, y=w47) -> (x*y=w43:dbl[])
              n39 = Multiply(x=w44, y=w45) -> (x*y=w42:dbl[])
              n40 = Compound Arithmetic op=ADD(w43, w42, w41) -> (w39:dbl[])
              n41 = Subtract(x=w39, y=w34) -> (x-y=w38:dbl[])
              n42 = global read "G_SEN.vi" "lane_thresh"() -> (w37:dbl)
              n43 = Absolute Value(x=w38) -> (abs(x)=w36:dbl[])
              n44 = Less Or Equal?(x=w37, y=w36) -> (x <= y?=w29:bool[])
              n45 = Not(x=w29) -> (.not. x?=w28:bool[])
              n46 = Boolean To (0,1)(Boolean=w29) -> (0, 1=w35:i16[])
              n47 = Boolean To (0,1)(Boolean=w28) -> (0, 1=w27:i16[])
              n48 = Build Cluster Array(w35, w34, w33, w32, w31) -> (w30:T3)
              n49 = To Long Integer(number=w27) -> (32bit integer=w26:i32[])
              n50 = Sort 1D Array(array=w30) -> (sorted array=w24:T3)
              n51 = Add Array Elements(numeric array=w26) -> (sum=w25:i32)
              n52 = local read "xsensor"() -> (w9:T1)
              n53 = for {
                N: w25 -> [_]
                tunnel: w24 -> [w55] mode=indexing
                tunnel: [w54] -> w15 mode=indexing
                tunnel: [w53] -> w14 mode=indexing
                tunnel: [w52] -> w23 mode=indexing
                tunnel: [w51] -> w22 mode=indexing
                n54 = Unbundle(w55) -> ("element"=w54:dbl, "element"=w53:dbl, "element"=w52:dbl, "element"=w51:dbl)  [unwired: 1 out]
              }
              n55 = Unbundle By Name(w9) -> ("x"=w16:dbl, "y"=w17:dbl, "h"=w18:dbl)
              n56 = Negate(x=w18) -> (-x=w19:dbl)
              n57 = call "rotm_mimo.vi"("angle[rad]"=w19, "reverse"=TRUE, "y0"=w17, "x0"=w16, "y"=w14, "x"=w15) -> ("Y"=w12:dbl[], "X"=w13:dbl[])  [unwired: 2 in, 2 out]
              n58 = Build Array(w13, w12, w23, w22) -> (w21:dbl[][])
              n59 = Transpose 2D Array(2D array=w21) -> (transposed array=w50:dbl[][])
            }
          }
          "sensor_out" <- w2
          n60 = Build Array (concatenate)(w8, w2) -> (→"lane_log_out":dbl[][])
        }
        frame #1 {
          n61 = flat-sequence {
            frame #0 {
              n62 = global read "G_NAV.vi" "M6006"() -> (w104:T2)
              n63 = local read "lane_log_out"() -> (w100:dbl[][])
              n64 = Unbundle By Name(w104) -> ("lcc[1]"=w103:dbl, "lcc[0]"=w102:dbl, "attitude[2]"=w101:dbl)
              n65 = Negate(x=w101) -> (-x=w108:dbl)
              n66 = Index Array(array=w100, index (col) #1=0 ("disabled index (col)")) -> (element #1=w110:dbl[], element #2=w111:dbl[])  [unwired: 3 in]
              n67 = call "rotm_mimo.vi"("angle[rad]"=w108, "reverse"=FALSE, "y0"=w102, "x0"=w103, "y"=w111, "x"=w110) -> ("Y"=→"Y":dbl[], "X"=→"X":dbl[])  [unwired: 2 in, 2 out]
            }
            frame #1 {
              n68 = disable-structure shown="Enabled" {
                frame Enabled {
                  n69 = local read "lane_M_out"() -> (w116:dbl[])
                  n70 = Index Array(array=w116, index=1) -> (element=w118:dbl)
                  n71 = Absolute Value(x=w118) -> (abs(x)=w117:dbl)
                  n72 = Multiply(x=w117, y=2.0) -> (x*y=w121:dbl)
                  n73 = Reciprocal(x=w121) -> (1/x=w120:dbl)
                  n74 = Multiply(x=0.05, y=w120) -> (x*y=w115:dbl)
                  n75 = local read "X"() -> (w139:dbl[])
                  n76 = local read "Y"() -> (w140:dbl[])
                  n77 = Max & Min(x=w115, y=15.0) -> (max(x,y)=w113:dbl)  [unwired: 1 out]
                  n78 = Square(x=w139) -> (x^2=w137:dbl[])
                  n79 = Square(x=w140) -> (x^2=w138:dbl[])
                  n80 = Square(x=w113) -> (x^2=w112:dbl)
                  n81 = Add(x=w138, y=w137) -> (x+y=w136:dbl[])
                  n82 = Greater?(x=w136, y=w112) -> (0:w128:bool[])
                  n83 = Not(x=w128) -> (.not. x?=w131:bool[])
                  n84 = Boolean To (0,1)(Boolean=w128) -> (0, 1=w129:i16[])
                  n85 = Boolean To (0,1)(Boolean=w131) -> (0, 1=w132:i16[])
                  n86 = local read "X"() -> (w127:dbl[])
                  n87 = local read "Y"() -> (w126:dbl[])
                  n88 = To Long Integer(number=w132) -> (32bit integer=w133:i32[])
                  n89 = Build Cluster Array(w129, w127, w126) -> (w130:T4)
                  n90 = Add Array Elements(numeric array=w133) -> (sum=w134:i32)
                  n91 = Sort 1D Array(array=w130) -> (sorted array=w135:T4)
                  n92 = for {
                    N: w134 -> [_]
                    tunnel: w135 -> [w143] mode=indexing
                    tunnel: [w142] -> w125 mode=indexing
                    tunnel: [w141] -> w124 mode=indexing
                    n93 = Unbundle(w143) -> ("Real Matrix Element"=w142:dbl, "Real Matrix Element"=w141:dbl)  [unwired: 1 out]
                  }
                  n94 = local write "X"(w125) -> ()
                  n95 = local write "Y"(w124) -> ()
                }
                frame Disabled {
                }
              }
            }
            frame #2 {
              n96 = local read "Y"() -> (w148:dbl[])
              n97 = Array Size(array=w148) -> (size(s)=w147:i32)
              "size" <- w147
              n98 = Greater Or Equal?(x=w147, y=10) -> (x >= y?=w146:bool)
              n99 = case shown="True" w146 {
                tunnel: [w152 w176] -> w144
                frame False {
                  n100 = local read "lane_M_out"() -> (w154:dbl[])
                  n101 = Index Array(array=w154, index=0) -> (element=w151:dbl)
                  n102 = Multiply(x=w151, y=0.8) -> (x*y=w149:dbl)
                  n103 = Replace Array Subset(array=w154, new element=w149, index=0) -> (w152:dbl[])
                }
                frame True {
                  n104 = local read "Y"() -> (w165:dbl[])
                  n105 = local read "X"() -> (w166:dbl[])
                  n106 = flat-sequence {
                    tunnel: w165 -> [w209]
                    tunnel: w166 -> [w206]
                    tunnel: [w202] -> w175
                    tunnel: [w201] -> w157
                    frame #0 {
                      n107 = Multiply(x=w209, y=w209) -> (x*y=w212:dbl[])
                      n108 = Multiply(x=w206, y=w209) -> (x*y=w208:dbl[])
                      n109 = Add Array Elements(numeric array=w206) -> (sum=w205:dbl)
                      n110 = Multiply(x=w209, y=w212) -> (x*y=w223:dbl[])
                      n111 = Multiply(x=w206, y=w212) -> (x*y=w211:dbl[])
                      n112 = Add Array Elements(numeric array=w208) -> (sum=w207:dbl)
                      n113 = Multiply(x=w209, y=w223) -> (x*y=w225:dbl[])
                      n114 = Add Array Elements(numeric array=w211) -> (sum=w210:dbl)
                      n115 = Array Size(array=w209) -> (size(s)=w219:i32)
                      n116 = Add Array Elements(numeric array=w225) -> (sum=w224:dbl)
                      n117 = Add Array Elements(numeric array=w209) -> (sum=w220:dbl)
                      n118 = Add Array Elements(numeric array=w223) -> (sum=w222:dbl)
                      n119 = Add Array Elements(numeric array=w212) -> (sum=w221:dbl)
                      n120 = To Double Precision Float(number=w219) -> (double precision float=w218:dbl)
                      n121 = Build Array(w210, w207, w205) -> (w203:dbl[])
                      n122 = Build Array(w221, w220, w218) -> (w215:dbl[])
                      n123 = Build Array(w224, w222, w221) -> (w217:dbl[])
                      n124 = Build Array(w222, w221, w220) -> (w216:dbl[])
                      n125 = Build Array(w217, w216, w215) -> (w214:dbl[][])
                      n126 = call-poly <vilib>:"Array To Matrix.vi"("Real 2D Array"=w214) -> ("Real Matrix"=w213:T5)
                      n127 = call-poly <vilib>:"Inverse Matrix.vi"("Input Matrix"=w213) -> ("error"=w201:i32, "Inverse Matrix"=w204:T5)  [unwired: 1 in]
                      n128 = call-poly <vilib>:"A x B.vi"("Vector"=w203, "A"=w204) -> ("A x Vector"=w202:dbl[])  [unwired: 1 out]
                    }
                  }
                  n129 = local read "lane_M_out"() -> (w158:dbl[])
                  n130 = Build Array (concatenate)(1.0, w175) -> (w161:dbl[])
                  n131 = Subtract(x=w161, y=w158) -> (x-y=w173:dbl[])
                  n132 = Absolute Value(x=w173) -> (abs(x)=w172:dbl[])
                  n133 = Index Array(array=w172, index #1=1 ("index")) -> (element #1=w170:dbl, element #2=w169:dbl)  [unwired: 1 in]
                  n134 = Add(x=w170, y=w169) -> (x+y=w168:dbl)
                  n135 = Index Array(array=w158, index=0) -> (element=w163:dbl)
                  n136 = Less?(x=w168, y="thresh") -> (x < y?=w160:bool)
                  n137 = Not Equal To 0?(x=w163) -> (x != 0?=w159:bool)
                  n138 = Equal To 0?(x=w157) -> (x = 0?=w156:bool)
                  n139 = Compound Arithmetic op=AND(w160, w159, w156) -> (w162:bool)
                  n140 = disable-structure shown="Enabled" {
                    disable-tunnel: [w179 w198] -> w176
                    disable-tunnel: w161 -> [w178 w199]
                    disable-tunnel: w162 -> [w177 w200]
                    disable-tunnel: w158 -> [_ w197]
                    frame Disabled {
                      n141 = case shown="False" w177 {
                        tunnel: [w184 w196] -> w179
                        tunnel: w178 -> [w190 w196]
                        frame False {
                          n142 = disable-structure shown="Enabled" {
                            disable-tunnel: w190 -> [w194 w195 _]
                            disable-tunnel: [w191 w195 _] -> w185
                            frame Disabled {
                              n143 = Replace Array Subset(array=w194, new element=0.0 ("new element/subarray"), index=0) -> (w191:dbl[])
                            }
                            frame Disabled {
                            }
                            frame Enabled {
                            }
                          }
                          n144 = local read "Lane_M"() -> (w183:dbl[])
                          n145 = Index Array(array=w183, index=0) -> (element=w188:dbl)
                          n146 = Replace Array Subset(array=w183, new element=0.8 ("new element/subarray"), index=0) -> (w180:dbl[])
                          n147 = Equal?(x=w188, y=1.0) -> (x = y?=w186:bool)
                          n148 = Select(t=w180, s=w186, f=w185) -> (s? t:f=w184:dbl[])
                        }
                        frame True {
                        }
                      }
                    }
                    frame Enabled {
                      n149 = Select(t=w199, s=w200, f=w197) -> (s? t:f=w198:dbl[])
                    }
                  }
                }
              }
              "lane_I_out" <- w144
            }
          }
        }
      }
    }
  }
